vi "TcA06-005_MissingAbstractMethod.vi"(1 "Input buffer":T3="1", 3 "Invocation info":T2, 5 "error in (no error)":errorcluster, 6 "Add log to result?":bool) -> (16 "Test Data":T1 {"Numeric Measurement" format="%.2f"}, 19 "error out":errorcluster)   [LabVIEW 2009]
doc: "Test case template."
uses:
  Shared/Support_InputBuffer.ctl
  Shared/Support_InvocationInfo.ctl
  Shared/Support_TestData.ctl
  TestClasses/G#BaseClass1_class/G#BaseClass1.lvclass
  TestClasses/G#SubClass1_class/G#SubClass1.lvclass
  <vilib>/addons/_AddQ/G#Object/G#Object.lvclass
panel:
  in  "Test name":string="TcA06-005 Missing Abstract Method"
  out "Test result":bool
  out "Result":string
  # "Verify that a missing abstract method generates an error."
  # "Sub test case"
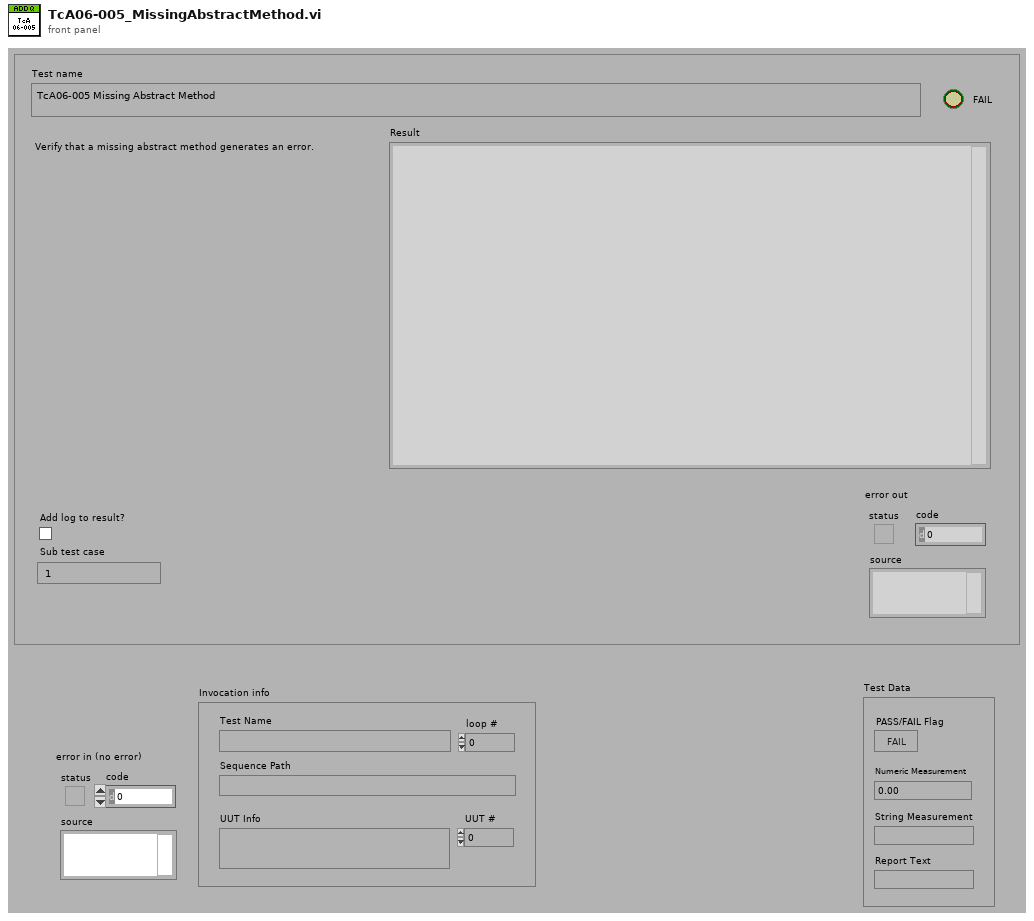
[diagram p1: front panel]
types:
  T1 = typedef "Support_TestData.ctl" = cluster{"PASS/FAIL Flag":bool, "Numeric Measurement":dbl, "String Measurement":string, "Report Text":string}
  T2 = typedef "Support_InvocationInfo.ctl" = cluster{"UUT #":i32, "loop #":i32, "UUT Info":string, "Test Name":string, "Sequence Path":path}
  T3 = typedef "Support_InputBuffer.ctl" = string
  T4 = typedef "Support_ResultType.ctl" = cluster{"Pass":bool, "Comment":string, "MeasurementValue":dbl}
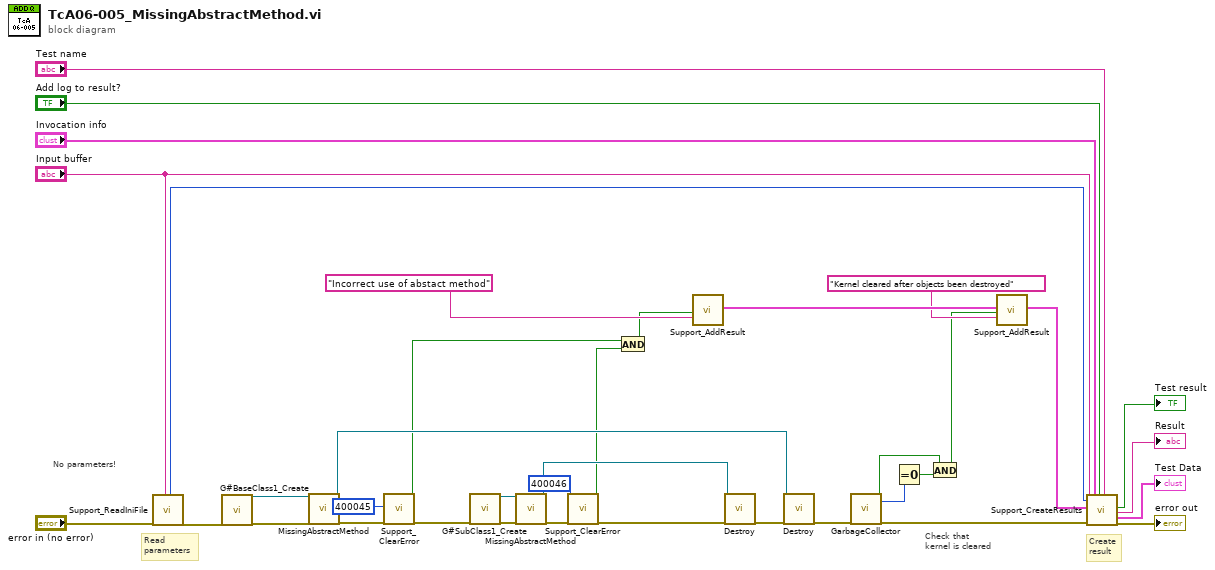
[diagram p0: block diagram]
diagram:
  # "Check that\nkernel is cleared"
  # "No parameters!"
  # "Create\nresult"
  # "Read\nparameters"
  n1 = call "Support_ReadIniFile.vi"("error in (no error)"="error in (no error)", "Sub test case"="Input buffer") -> ("Timer start"=w28:u32, "error out"=w22:errorcluster)  [unwired: 10 in, 6 out]
  n2 = call "G#BaseClass1_Create.vi"("error in (no error)"=w22) -> ("reference out"=w14:refnum<class "G#BaseClass1.lvclass">, "error out"=w11:errorcluster)  [unwired: 16 in, 1 out]
  n3 = call-dynamic "MissingAbstractMethod.vi"("reference in"=w14, "error in (no error)"=w11) -> ("reference out"=w13:refnum<class "G#BaseClass1.lvclass">, "error out"=w15:errorcluster)  [unwired: 16 in]
  n4 = call "Support_ClearError.vi"("code"=400045, "error in (no error)"=w15) -> ("Cleared?"=w2:bool, "error out"=w12:errorcluster)  [unwired: 16 in]
  n5 = call "G#SubClass1_Create.vi"("error in (no error)"=w12) -> ("reference out"=w9:refnum<class "G#SubClass1.lvclass">, "error out"=w10:errorcluster)  [unwired: 16 in, 1 out]
  n6 = call-dynamic "MissingAbstractMethod.vi"("reference in"=w9, "error in (no error)"=w10) -> ("reference out"=w4:refnum<class "G#SubClass1.lvclass">, "error out"=w6:errorcluster)  [unwired: 16 in]
  n7 = call "Support_ClearError.vi"("code"=400046, "error in (no error)"=w6) -> ("Cleared?"=w3:bool, "error out"=w5:errorcluster)  [unwired: 16 in]
  n8 = And(x=w2, y=w3) -> (x .and. y?=w1:bool)
  n9 = call "Support_AddResult.vi"("Pass"=w1, "Comment"="Incorrect use of abstact method") -> ("Results out"=w25:T4[])  [unwired: 17 in]
  n10 = call-dynamic "Destroy.vi"("reference in"=w4, "error in (no error)"=w5) -> ("error out"=w8:errorcluster)  [unwired: 16 in, 1 out]
  n11 = call-dynamic "Destroy.vi"("reference in"=w13, "error in (no error)"=w8) -> ("error out"=w16:errorcluster)  [unwired: 16 in, 1 out]
  n12 = call <vilib>:"GarbageCollector.vi"("error in (no error)"=w16) -> ("OK"=w19:bool, "# of objects killed"=w21:i32, "error out"=w27:errorcluster)  [unwired: 16 in]
  n13 = Equal To 0?(x=w21) -> (x = 0?=w20:bool)
  n14 = And(x=w19, y=w20) -> (x .and. y?=w18:bool)
  n15 = call "Support_AddResult.vi"("Results in"=w25, "Pass"=w18, "Comment"="Kernel cleared after objects been destroyed") -> ("Results out"=w24:T4[])  [unwired: 16 in]
  n16 = call "Support_CreateResults.vi"("Sub test case"="Input buffer", "Timer start"=w28, "Results"=w24, "error in (no error)"=w27, "Invocation info"="Invocation info", "Add log to result?"="Add log to result?", "Test name"="Test name") -> ("Pass/fail flag"=→"Test result":bool, "Result"=→"Result":string, "Test Data"=→"Test Data":T1, "error out"=→"error out":errorcluster)  [unwired: 9 in]
